vi "SetSettings.vi"(8 "error in (no error)":errorcluster, 10 "Variant":variant, 11 "ChromaPowerSupplyModel in":refnum<class "ChromaPowerSupplyModel.lvclass">) -> (0 "error out":errorcluster, 3 "ChromaPowerSupplyModel Out":refnum<class "ChromaPowerSupplyModel.lvclass">)   [LabVIEW 2018, in "AcPwrPlugins.lvlib" / "ChromaPowerSupplyModel.lvclass"]
doc: "This VI sets the instruments properties."
uses:
  ChromaPowerSupplyModel.lvclass
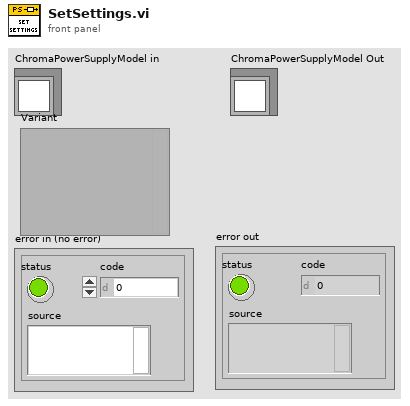
[diagram p1: front panel]
types:
  T1 = typedef "AcPwrPlugins.lvlib/ChromaPowerSupply.lvclass/Measurements.ctl" = cluster{"Handle":string, "Name":string, "Enabled":bool, "Measurement Value":dbl, "btnMeasFetch":bool, "ProtectionStatusString":string, "Measurement Type":enum16{"Voltage", "Current", "Power"}}[]
  T2 = typedef "AcPwrPlugins.lvlib/ChromaPowerSupply.lvclass/Device(s)Settings.ctl" = cluster{"Phases":cluster{"Handle":string, "Instrument Options":string, "id query (T)":bool, "reset device (T)":bool, "Timing":cluster{"TimingOn":enum16{""}, "Hours":u32, "Minutes":u32, "Seconds":dbl, "CutoffVoltage":dbl}, "Connected":bool, "Output Mode":enum16{"Voltage (DC)", "Current (DC)"}, "Voltage":dbl, "Current":dbl, "High Voltage Limit":dbl, "High Current Limit":dbl, "Power Protect":dbl, "Current Protect":dbl, "Voltage Protect":dbl, "Low Current Limit":dbl, "Low Voltage Limit":dbl, "Current Slew Rate":dbl, "Voltage Slew Rate":dbl, "Current Slew Infinite?":bool}[], "MeasName":string}
  T3 = typedef "AcPwrShared.lvlib/Database Settings.ctl" = cluster{"Data Source":string, "ICDAS to Model Table":string, "Model to ICDAS Table":string}
  T4 = cluster{"Device Settings":T2, "Database Settings":T3}
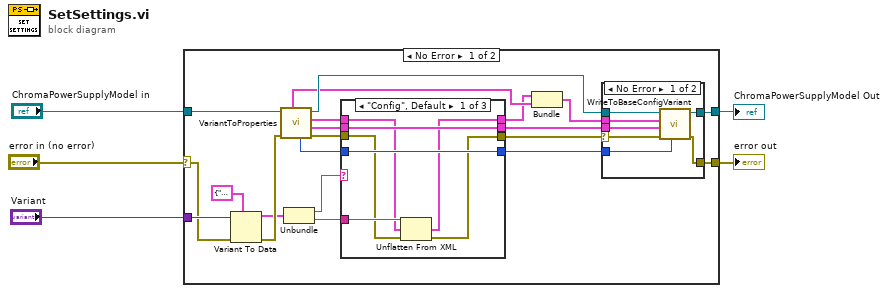
[diagram p0: block diagram]
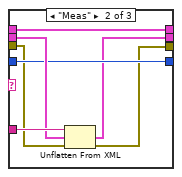
[diagram p3: hidden frame]
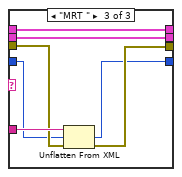
[diagram p4: hidden frame]
diagram:
  n1 = case shown="No Error" "error in (no error)" {
    selector: "error in (no error)" -> [w25 w57]
    tunnel: "ChromaPowerSupplyModel in" -> [w23 w58]
    tunnel: [w11 w58] -> w3
    tunnel: [w10 w57] -> w2
    tunnel: "Variant" -> [w26 _]
    frame No Error {
      n2 = Variant To Data(error in=w25, type=cluster{string, string} {"", ""}, Variant=w26) -> (data=w21:cluster{string, string}, error out=w22:errorcluster)
      n3 = call "VariantToProperties.vi"("error in (no error)"=w22, "ChromaPowerSupplyModel in"=w23) -> ("error out"=w18:errorcluster, "Measurements"=w19:T1, "Device Settings"=w20:T2, "ChromaPowerSupplyModel out"=w14:refnum<class "ChromaPowerSupplyModel.lvclass">, "Measurement Refresh Time (ms)"=w15:u32, "Database Settings"=w8:T3)  [unwired: 4 in]
      n4 = Unbundle(w21) -> (w17:string, w16:string)
      n5 = case shown="\"Config\", Default" w17 {
        tunnel: w20 -> [w36 w46 w54]
        tunnel: w19 -> [w39 w48 w53]
        tunnel: w18 -> [w40 w45 w55]
        tunnel: w16 -> [w41 w49 w56]
        tunnel: [w38 w46 w54] -> w7
        tunnel: [w39 w43 w53] -> w13
        tunnel: w15 -> [w42 w47 w52]
        tunnel: [w42 w47 w50] -> w9
        tunnel: [w37 w44 w51] -> w12
        frame "Config", Default {
          n6 = Unflatten From XML(xml string=w41, type=w36, error in (no error)=w40) -> (value=w38:T2, error out=w37:errorcluster)
        }
        frame "Meas" {
          n7 = Unflatten From XML(xml string=w49, type=w48, error in (no error)=w45) -> (value=w43:T1, error out=w44:errorcluster)
        }
        frame "MRT " {
          n8 = Unflatten From XML(xml string=w56, type=w52, error in (no error)=w55) -> (value=w50:u32, error out=w51:errorcluster)
        }
      }
      n9 = Bundle("Device Settings"=w7, "Database Settings"=w8) -> (w6:T4)  [unwired: 1 in]
      n10 = case shown="No Error" w12 {
        selector: w12 -> [w32 w34]
        tunnel: w14 -> [w33 w35]
        tunnel: w6 -> [w28 _]
        tunnel: w13 -> [w27 _]
        tunnel: [w31 w35] -> w11
        tunnel: [w30 w34] -> w10
        tunnel: w9 -> [w29 _]
        frame No Error {
          n11 = call-dynamic "WriteToBaseConfigVariant.vi"("Measurement Refresh Time (ms)"=w29, "error in (no error)"=w32, "Meas"=w27, "Config"=w28, "ChromaPowerSupplyModel in"=w33) -> ("error out"=w30:errorcluster, "ChromaPowerSupplyModel out"=w31:refnum<class "ChromaPowerSupplyModel.lvclass">)  [unwired: 5 in]
        }
        frame Error {
        }
      }
    }
    frame Error {
    }
  }
  "error out" <- w2
  "ChromaPowerSupplyModel Out" <- w3
